vi "Save Recall List Program.vi"(8 "error in (no error)":errorcluster, 9 "List Number (0)":i32 min=0 max=9 format="%#_0f", 10 "Save Recall List File (0:Save)":u16(ring) items=["Save", "Recall"], 11 "VISA resource name":refnum<visa-resource-name>) -> (0 "error out":errorcluster, 3 "VISA resource name out":refnum<visa-resource-name>)   [LabVIEW 2021, in "BK Precision 9200 Series.lvlib"]
doc: "Saves or recalls list programs to or from internal memory of the instrument. When using this vi to save a list program, all list parameters and configurations will be saved to the location specified by <b>List Number</b>.\nBefore saving a list program, run the <b>Configure List Parameters.vi</b> and <b>Configure List Repeat.vi</b> first and in order."
uses:
  <instrlib>/BK Precision 9200 Series/BK Precision 9200 Series.lvlib
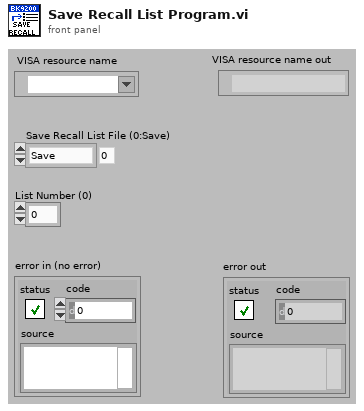
[diagram p1: front panel]
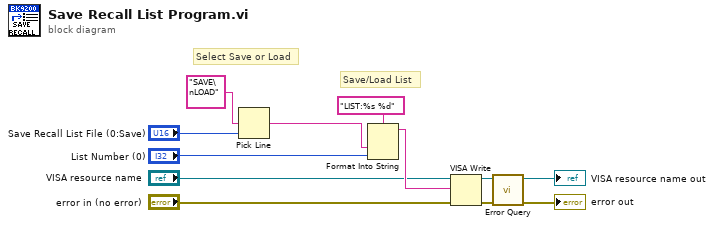
[diagram p0: block diagram]
diagram:
  # "Select Save or Load"
  # "Save/Load List"
  n1 = Pick Line(multi-line string="SAVE\nLOAD", line index="Save Recall List File (0:Save)") -> (output string=w1:string)  [unwired: 1 in]
  n2 = Format Into String(format string="LIST:%s %d", w1, "List Number (0)") -> (resulting string=w8:string)  [unwired: 2 in, 1 out]
  n3 = VISA Write(VISA resource name="VISA resource name", write buffer=w8, error in (no error)="error in (no error)") -> (VISA resource name out=w12:refnum<visa-resource-name>, error out=w11:errorcluster)  [unwired: 1 out]
  n4 = call <instrlib>:"Error Query.vi"("error in (no error)"=w11, "VISA resource name"=w12) -> ("error out"=→"error out":errorcluster, "VISA resource name out"=→"VISA resource name out":refnum<visa-resource-name>)  [unwired: 6 in, 2 out]
